vi "Get Prompt Message.vi"(0 "VISA resource name":refnum<visa-resource-name>, 7 "Step Number (1 - 2000)":i32 min=0 max=60, 11 "error in (no error)":errorcluster) -> (4 "VISA resource name out":refnum<visa-resource-name>, 8 "Step Prompt":string, 15 "error out":errorcluster)   [LabVIEW 2012, in "Associated Research 78XX Series.lvlib"]
doc: "LP <step number>?\nLists the prompt that has been created for of one of the steps of the file within active memory (RAM)."
uses:
  <instrlib>/Associated Research 78XX Series/Associated Research 78XX Series.lvlib
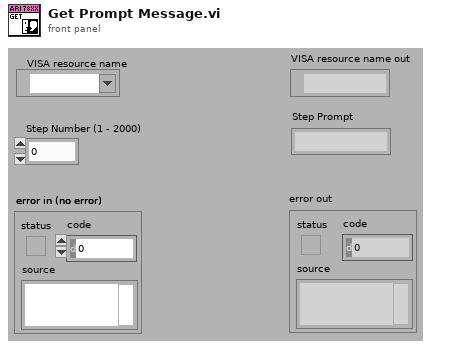
[diagram p1: front panel]
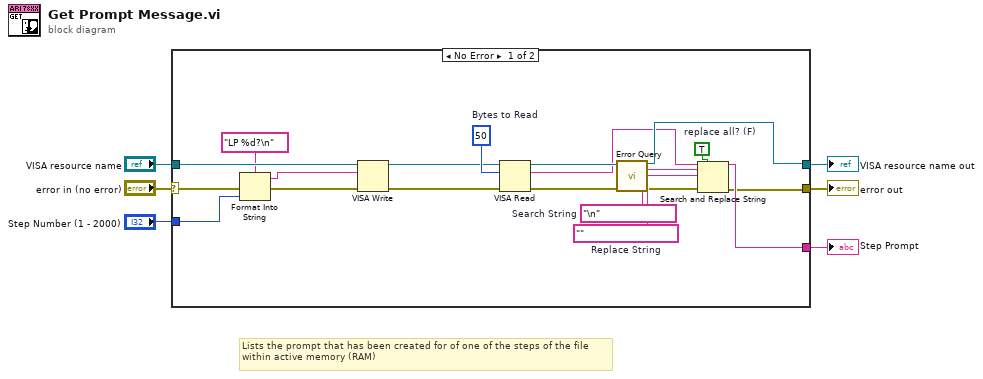
[diagram p0: block diagram]
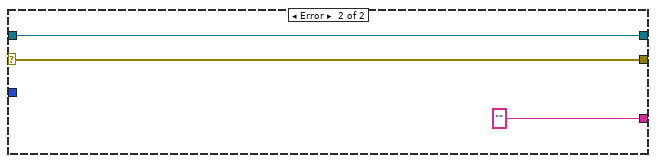
[diagram p2: hidden frame]
diagram:
  # "Lists the prompt that has been created for of one of the steps of the file within active memory (RAM)"
  n1 = case shown="No Error" "error in (no error)" {
    selector: "error in (no error)" -> [w23 w28]
    tunnel: [w16 w28] -> w5
    tunnel: [w14 w27] -> w3
    tunnel: "VISA resource name" -> [w25 w27]
    tunnel: "Step Number (1 - 2000)" -> [w21 _]
    tunnel: [w18 "" ("read buffer")] -> w1
    frame No Error {
      w11 = u32 50  # Bytes to Read
      w17 = TRUE  # replace all? (F)
      w19 = ""  # Replace String
      w20 = "\n"  # Search String
      n2 = Format Into String(format string="LP %d?\n" ("\"False\" Command"), error in=w23, w21) -> (resulting string=w7:string, error out=w22:errorcluster)  [unwired: 1 in]
      n3 = VISA Write(VISA resource name=w25, write buffer=w7, error in (no error)=w22) -> (VISA resource name out=w10:refnum<visa-resource-name>, error out=w9:errorcluster)  [unwired: 1 out]
      n4 = VISA Read(VISA resource name=w10, byte count=w11, error in (no error)=w9) -> (VISA resource name out=w12:refnum<visa-resource-name>, read buffer=w8:string, error out=w13:errorcluster)  [unwired: 1 out]
      n5 = call <instrlib>:"Error Query.vi"("VISA resource name"=w12, "error in (no error)"=w13) -> ("VISA resource name out"=w14:refnum<visa-resource-name>, "error out"=w15:errorcluster)  [unwired: 10 in, 2 out]
      n6 = Search and Replace String(replace all?=w17, input string=w8, search string=w20, replace string=w19, error in=w15) -> (result string=w18:string, error out=w16:errorcluster)  [unwired: 3 in, 2 out]
    }
    frame Error {
    }
  }
  "error out" <- w5
  "VISA resource name out" <- w3
  "Step Prompt" <- w1
